vi "Find_SLM.vi"(9 "Picture Control":refnum<vi>, 10 "Full Screen":bool, 11 "Monitor":i32) -> (1 "Monitor Picture":picture, 2 "Selected Monitor is 1024x768":bool, 3 "Window Rect":i16[](array[numeric]), 5 "Sensible Default Monitor (BNS)":i32)   [LabVIEW 2015]
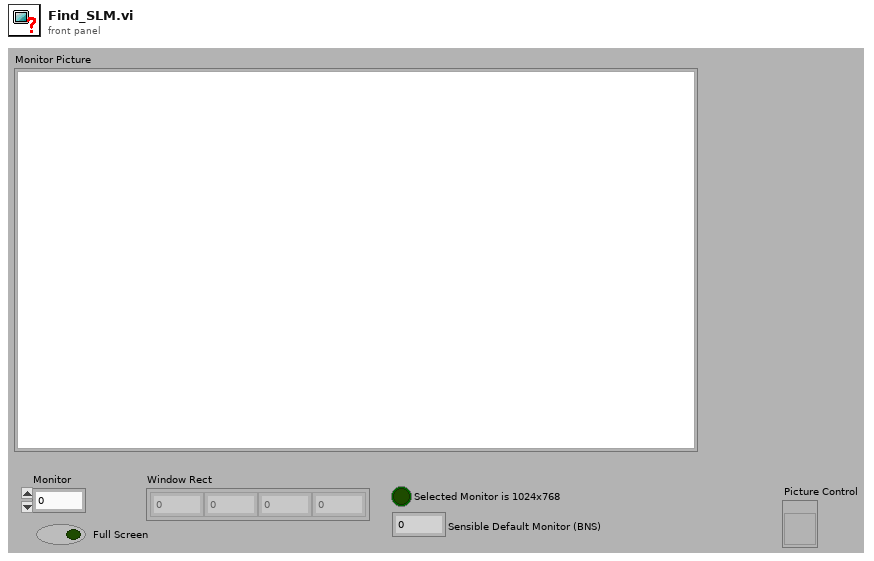
[diagram p1: front panel]
types:
  T1 = typedef "LVAllMonitorsDisplayTypeDef.ctl" = cluster{"Bounds":cluster{"Left":i16, "Top":i16, "Right":i16, "Bottom":i16}, "Depth":i16}[]
  T2 = cluster{"horizontal":enum16{"left", "center", "right"}, "vertical":enum16{"top", "center", "bottom"}}
  T3 = cluster{"Font Name:":string, "Size":i16, "Strikeout?":bool, "Italic?":bool, "Underline?":bool, "Outline?":bool, "Shadow?":bool, "Bold?":bool}
  T4 = enum16{"User-specified Font", "Application Font", "System Font", "Dialog Font"}
  T5 = cluster{"Width":i16, "Style":enum32{"Solid", "Dash", "Dot", "DashDot", "DashDotDot"}}
  T6 = cluster{"Left":i16, "Top":i16, "Right":i16, "Bottom":i16}
  T7 = typedef "LVBoundsTypeDef.ctl" = cluster{"Width":u32, "Height":u32}
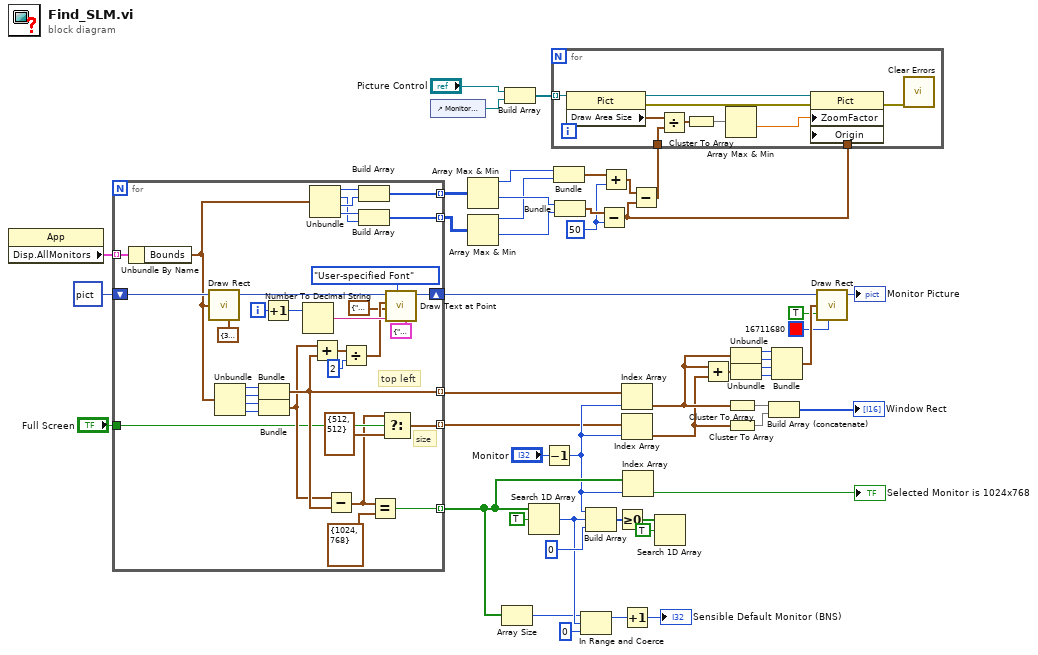
[diagram p0: block diagram]
diagram:
  w39 = i16 50 ("Left")
  n1 = property class="App"() -> ("Disp.AllMonitors"=w49:T1)  [unwired: 2 in, 2 out]
  n2 = for {
    tunnel: w49 -> [w82] mode=indexing
    shift-right: [w66] -> w35
    shift-left: picture data[5B] ("new picture") -> [w81]
    tunnel: [w75] -> w47 mode=indexing
    tunnel: [w74] -> w46 mode=indexing
    tunnel: [w57] -> w33 mode=indexing
    tunnel: [w56] -> w9 mode=indexing
    tunnel: "Full Screen" -> [w53]
    tunnel: [w51] -> w4 mode=indexing
    i -> [w64]
    # "size"
    # "top left"
    n3 = Unbundle By Name(w82) -> ("Bounds"=w65:T6)
    n4 = call <vilib>:"Draw Rect.vi"("picture"=w81, "rect"=w65, "pen"=T5 {"Width"=3, "Style"=enum."Solid"}) -> ("new picture"=w67:picture)  [unwired: 6 in]
    n5 = Unbundle(w65) -> ("Left"=w73:i16, "Top"=w72:i16, "Right"=w71:i16, "Bottom"=w70:i16)
    n6 = Bundle("Left"=w73, "Top"=w72) -> (w57:cluster{"Left":i16, "Top":i16})  [unwired: 1 in]
    n7 = Bundle("Right"=w71, "Bottom"=w70) -> (w54:cluster{"Right":i16, "Bottom":i16})  [unwired: 1 in]
    n8 = Increment(x=w64) -> (x+1=w55:i32)
    n9 = Number To Decimal String(number=w55) -> (decimal integer string=w63:string)  [unwired: 1 in]
    n10 = Unbundle(w65) -> ("Left"=w79:i16, "Top"=w76:i16, "Right"=w78:i16, "Bottom"=w77:i16)
    n11 = Add(x=w54, y=w57) -> (x+y=w69:cluster{i16, i16})
    n12 = Subtract(x=w54, y=w57) -> (x-y=w50:cluster{i16, i16})
    n13 = Divide(x=w69, y=i16 2 ("Left")) -> (x/y=w60:cluster{dbl, dbl})
    n14 = Build Array(w79, w78) -> (w75:i16[])
    n15 = Build Array(w77, w76) -> (w74:i16[])
    n16 = Equal?(x=w50, y=cluster{i16, i16} {1024, 768}) -> (x = y?=w56:bool)
    n17 = Select(t=w50, s=w53, f=cluster{"Right":i16, "Bottom":i16} {"Right"=512, "Bottom"=512}) -> (s? t:f=w51:cluster{"Right":i16, "Bottom":i16})
    n18 = call <vilib>:"Draw Text at Point.vi"("[user-specified font]"=T3 {"Font Name:"="Arial", "Size"=400, "Strikeout?"=FALSE, "Italic?"=FALSE, "Underline?"=FALSE, "Outline?"=FALSE, "Shadow?"=FALSE, "Bold?"=TRUE}, "desired font(Application)"=T4."User-specified Font", "text"=w63, "alignment(left, top)"=T2 {"horizontal"=enum."center", "vertical"=enum."center"}, "origin"=w60, "picture"=w67) -> ("new picture"=w66:picture)  [unwired: 4 in, 1 out]
  }
  n19 = control-ref of="Monitor Picture"() -> (w14:refnum<vi>)
  n20 = Array Max & Min(array=w47) -> (max value=w42:i16, min value=w45:i16)  [unwired: 2 out]
  n21 = Array Max & Min(array=w46) -> (max value=w41:i16, min value=w44:i16)  [unwired: 2 out]
  n22 = Array Size(array=w9) -> (size(s)=w10:i32)
  n23 = Build Array("Picture Control", w14) -> (w13:refnum<vi>[])
  n24 = Search 1D Array(1D array=w9, element=TRUE) -> (index of element=w12:i32)  [unwired: 1 in]
  n25 = Decrement(x="Monitor") -> (x-1=w5:i32)
  n26 = Bundle(w42, w41) -> (w40:cluster{i16, i16})  [unwired: 1 in]
  n27 = Bundle(w45, w44) -> (w43:cluster{i16, i16})  [unwired: 1 in]
  n28 = In Range and Coerce(upper limit=w10, x=w12, lower limit=0) -> (coerced(x)=w8:i32)  [unwired: 1 out]
  n29 = Build Array(w5, w12, 0 ("index of element")) -> (w30:i32[])
  n30 = Subtract(x=w43, y=w39) -> (x-y=w36:cluster{i16, i16})
  n31 = Add(x=w40, y=w39) -> (x+y=w38:cluster{i16, i16})
  n32 = Greater Or Equal To 0?(x=w30) -> (x >= 0?=w28:bool[])
  n33 = Index Array(array=w33, index=w5) -> (element=w23:cluster{"Left":i16, "Top":i16})
  n34 = Index Array(array=w4, index=w5) -> (element=w3:cluster{"Right":i16, "Bottom":i16})
  n35 = Increment(x=w8) -> (x+1=→"Sensible Default Monitor (BNS)":i32)
  n36 = Index Array(array=w9, index=w5) -> (element=→"Selected Monitor is 1024x768":bool)
  n37 = Subtract(x=w38, y=w36) -> (x-y=w37:cluster{i16, i16})
  n38 = for {
    tunnel: w37 -> [w92]
    tunnel: w36 -> [w87]
    tunnel: w13 -> [w83] mode=indexing
    n39 = property on="Property Node" class="Pict"(reference=w83) -> (reference out=w86:refnum<vi>, error out=w85:errorcluster, "Draw Area Size"=w91:T7)  [unwired: 1 in]
    n40 = Divide(x=w91, y=w92) -> (x/y=w90:cluster{dbl, dbl})
    n41 = Cluster To Array(cluster=w90) -> (array=w89:dbl[])
    n42 = Array Max & Min(array=w89) -> (min value=w88:dbl)  [unwired: 3 out]
    n43 = property on="Property Node" class="Pict"(reference=w86, error in=w85, "ZoomFactor"=w88, "Origin"=w87) -> (error out=w84:errorcluster)  [unwired: 1 out]
    n44 = call <vilib>:"Clear Errors.vi"("error in (no error)"=w84) -> ()  [unwired: 5 in, 2 out]
  }
  n45 = Search 1D Array(1D array=w28, element=TRUE) -> ()  [unwired: 1 in, 1 out]
  n46 = Add(x=w23, y=w3) -> (x+y=w24:cluster{i16, i16})
  n47 = Cluster To Array(cluster=w23) -> (array=w1:i16[])
  n48 = Cluster To Array(cluster=w3) -> (array=w2:i16[])
  n49 = Unbundle(w23) -> ("Left"=w22:i16, "Top"=w21:i16)
  n50 = Unbundle(w24) -> (w20:i16, w19:i16)
  n51 = Build Array (concatenate)(w1, w2) -> (→"Window Rect":i16[])
  n52 = Bundle("Left"=w22, "Top"=w21, w20, w19) -> (w18:cluster{"Left":i16, "Top":i16, i16, i16})  [unwired: 1 in]
  n53 = call <vilib>:"Draw Rect.vi"("picture"=w35, "rect"=w18, "fill?(F)"=TRUE, "color(black)"=u32 16711680) -> ("new picture"=→"Monitor Picture":picture)  [unwired: 5 in]
